vi "Fc_to_define_CSstatus.vi"(6 "Class TCP in":T1, 7 "CS enable":bool, 8 "error in (no error)":errorcluster, 10 "CS enable":refnum<vi>, 11 "# Control?":refnum<vi>) -> (0 "error out":errorcluster, 3 "Class TCP out":T1)   [LabVIEW 2021]
doc: "This function defines the current status of the control system."
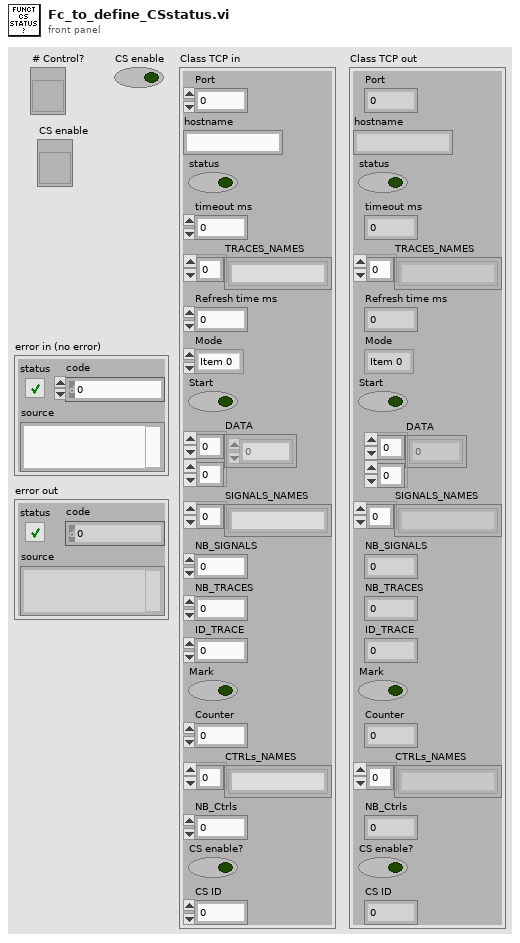
[diagram p1: front panel]
types:
  T1 = cluster{"Port":i32, "hostname":string, "status":bool, "timeout ms":i32, "TRACES_NAMES":string[], "Refresh time ms":i32, "Mode":enum32{"Item 0", "Item 1"}, "Start":bool, "DATA":sgl[][], "SIGNALS_NAMES":string[], "NB_SIGNALS":i32, "NB_TRACES":i32, "ID_TRACE":i32, "Mark":bool, "Counter":i32, "CTRLs_NAMES":string[], "NB_Ctrls":i32, "CS enable?":bool, "CS ID":i32}
  T2 = cluster{"TRACE_SIZE":i32, "CS_ID":i32, "TRACE ID":i32, "CMD":i32, "DATA(M)":i32}
  T3 = cluster{"timeout ms":i32, "remote port":u16, "Address":string}
  T4 = cluster{"SIZE":i32, " TRACE DATA":sgl[], "TRACE_SIZE":i32, "NB_TRACES":i32, "NB_TRACED_SIGNALS":i32, "NAMES TRACED SIGNALS":string[], "NAMES TRACES":string[], "CS STATUS":i32, "NB_CSs":i32, "NAMES CSs":string[], "DATA (M)":sgl[], "CMD":i32}
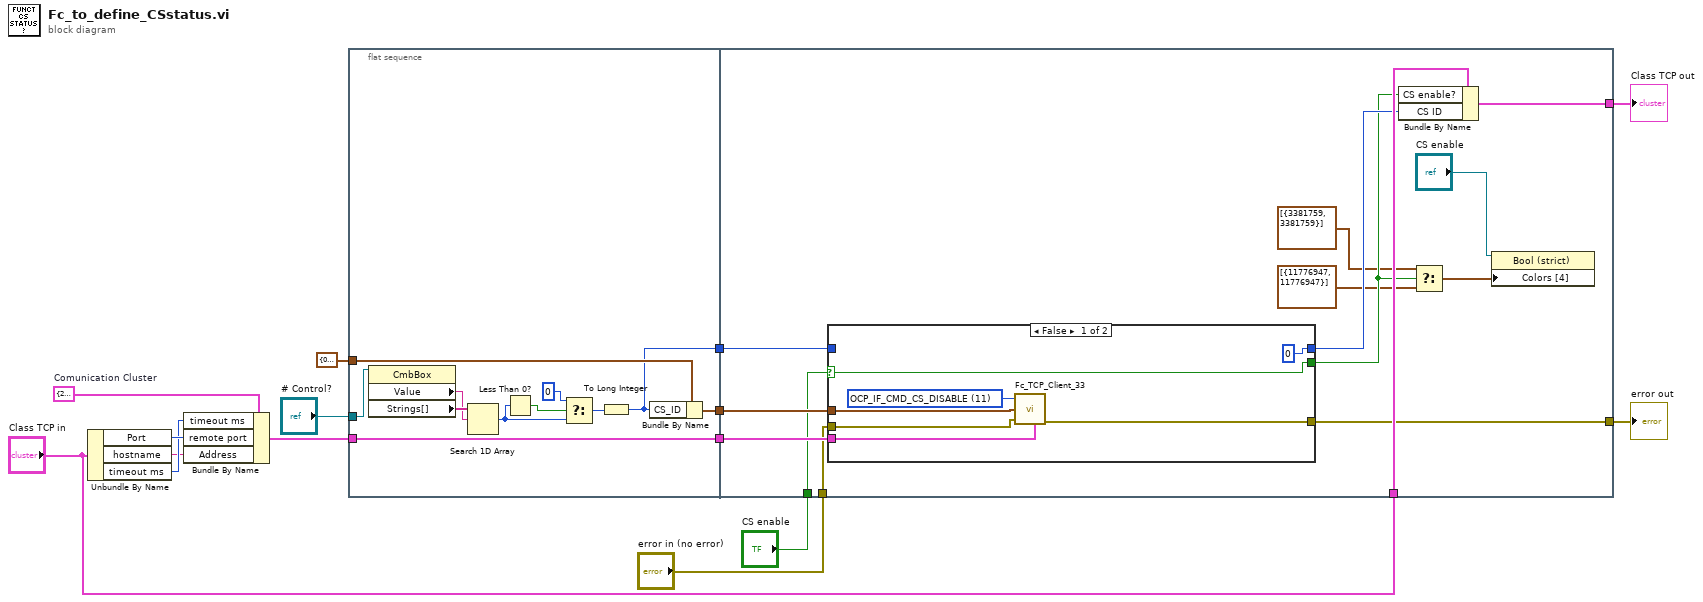
[diagram p0: block diagram]
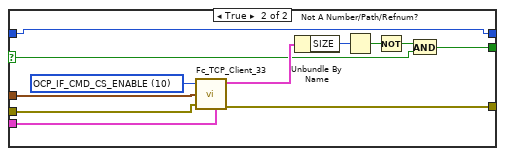
[diagram p2: hidden frame]
diagram:
  w12 = T3 {"timeout ms"=2000, "remote port"=8085, "Address"="127.0.0.1"}  # Comunication Cluster
  n1 = Unbundle By Name("Class TCP in") -> ("Port"=w6:i32, "hostname"=w4:string, "timeout ms"=w5:i32)
  n2 = Bundle By Name(cluster=w12, "timeout ms"=w5, "remote port"=w6, "Address"=w4) -> (w3:T3)
  n3 = flat-sequence {
    tunnel: T2 {"TRACE_SIZE"=0, "CS_ID"=0, "TRACE ID"=0, "CMD"=0, "DATA(M)"=0} ("Input Cluster") -> [w24]
    tunnel: w3 -> [w23]
    tunnel: [w23] -> w15
    tunnel: [w22] -> w14
    tunnel: [w17] -> w13
    tunnel: "# Control?" -> [w16]
    tunnel: w15 -> [w39]
    tunnel: w14 -> [w40]
    tunnel: "Class TCP in" -> [w38]
    tunnel: [w37] -> w7
    tunnel: w13 -> [w36]
    tunnel: "error in (no error)" -> [w30]
    tunnel: [w29] -> w10
    tunnel: "CS enable" -> [w28]
    frame #0 {
      n4 = property on="Property Node" class="CmbBox"(reference=w16) -> ("Value"=w25:string, "Strings[]"=w26:string[])  [unwired: 1 in, 2 out]
      n5 = Search 1D Array(1D array=w26, element=w25) -> (index of element=w20:i32)  [unwired: 1 in]
      n6 = Less Than 0?(x=w20) -> (x < 0?=w21:bool)
      n7 = Select(t=0, s=w21, f=w20) -> (s? t:f=w18:i32)
      n8 = To Long Integer(number=w18) -> (32bit integer=w17:i32)
      n9 = Bundle By Name(cluster=w24, "CS_ID"=w17) -> (w22:T2)
    }
    frame #1 {
      n10 = case shown="False" w28 {
        selector: w28 -> [w43 w54]
        tunnel: w39 -> [w47 w59]
        tunnel: w40 -> [w44 w56]
        tunnel: [w45 w57] -> w29
        tunnel: [w43 w53] -> w34
        tunnel: w36 -> [_ w52]
        tunnel: [0 w52] -> w35
        tunnel: w30 -> [w41 w48]
        frame False {
          w46 = 11 items=["OCP_IF_CMD_TRACE_READ", "OCP_IF_CMD_TRACE_RESET", "OCP_IF_CMD_TRACE_GET_SIZE", "OCP_IF_CMD_TRACE_SET_SIZE", "OCP_IF_CMD_TRACE_GET_NUMBER_SIGNALS", "OCP_IF_CMD_TRACE_GET_SIGNALS_NAMES", "OCP_IF_CMD_TRACE_GET_NUMBER_TRACES", "OCP_IF_CMD_TRACE_GET_TRACES_NAMES", "OCP_IF_CMD_TRACE_GET_ADDRESS", "OCP_IF_CMD_CS_STATUS", "OCP_IF_CMD_CS_ENABLE", "OCP_IF_CMD_CS_DISABLE", "OCP_IF_CMD_CS_CONTROLLER_IF", "OCP_IF_CMD_CS_HARDWARE_IF", "OCP_IF_CMD_CS_GET_NUMBER_CONTROLLERS", "OCP_IF_CMD_CS_GET_CONTROLLERS_NAMES", "OCP_IF_CMD_PLATFORM_ID", "OCP_IF_CMD_PLATFORM_IF", "OCP_IF_CMD_OPIL_UPDATE_MEASUREMENTS", "OCP_IF_CMD_OPIL_UPDATE_SIM_DATA", "OCP_IF_CMD_OPIL_RUN_CONTROL", "OCP_IF_CMD_OPIL_INITIALIZE_CONTROL", "OCP_IF_CMD_OPIL_GET_CONTROL", "OCP_IF_CMD_OPIL_GET_CONTROLLER_DATA", "OCP_IF_CMD_END"] ("CMD")
          n11 = call "Fc_TCP_Client_33.vi"("CMD"=w46, "Input Cluster"=w44, "error in (no error)"=w41, "Comunication Cluster"=w47) -> ("error out"=w45:errorcluster)  [unwired: 4 in, 2 out]
        }
        frame True {
          w58 = 10 items=["OCP_IF_CMD_TRACE_READ", "OCP_IF_CMD_TRACE_RESET", "OCP_IF_CMD_TRACE_GET_SIZE", "OCP_IF_CMD_TRACE_SET_SIZE", "OCP_IF_CMD_TRACE_GET_NUMBER_SIGNALS", "OCP_IF_CMD_TRACE_GET_SIGNALS_NAMES", "OCP_IF_CMD_TRACE_GET_NUMBER_TRACES", "OCP_IF_CMD_TRACE_GET_TRACES_NAMES", "OCP_IF_CMD_TRACE_GET_ADDRESS", "OCP_IF_CMD_CS_STATUS", "OCP_IF_CMD_CS_ENABLE", "OCP_IF_CMD_CS_DISABLE", "OCP_IF_CMD_CS_CONTROLLER_IF", "OCP_IF_CMD_CS_HARDWARE_IF", "OCP_IF_CMD_CS_GET_NUMBER_CONTROLLERS", "OCP_IF_CMD_CS_GET_CONTROLLERS_NAMES", "OCP_IF_CMD_PLATFORM_ID", "OCP_IF_CMD_PLATFORM_IF", "OCP_IF_CMD_OPIL_UPDATE_MEASUREMENTS", "OCP_IF_CMD_OPIL_UPDATE_SIM_DATA", "OCP_IF_CMD_OPIL_RUN_CONTROL", "OCP_IF_CMD_OPIL_INITIALIZE_CONTROL", "OCP_IF_CMD_OPIL_GET_CONTROL", "OCP_IF_CMD_OPIL_GET_CONTROLLER_DATA", "OCP_IF_CMD_END"] ("CMD")
          n12 = call "Fc_TCP_Client_33.vi"("CMD"=w58, "Input Cluster"=w56, "error in (no error)"=w48, "Comunication Cluster"=w59) -> ("Output cluster"=w55:T4, "error out"=w57:errorcluster)  [unwired: 4 in, 1 out]
          n13 = Unbundle By Name(w55) -> ("SIZE"=w51:i32)
          n14 = Not A Number/Path/Refnum?(number/path/refnum=w51) -> (NaN/Path/Refnum?=w50:bool)
          n15 = Not(x=w50) -> (.not. x?=w49:bool)
          n16 = And(x=w49, y=w54) -> (x .and. y?=w53:bool)
        }
      }
      n17 = Bundle By Name(cluster=w38, "CS enable?"=w34, "CS ID"=w35) -> (w37:T1)
      n18 = Select(t=cluster{u32, u32}[] [{3381759, 3381759}] ("Colors [4]"), s=w34, f=cluster{u32, u32}[] [{11776947, 11776947}] ("Colors [4]")) -> (s? t:f=w33:cluster{u32, u32}[])
      n19 = property on="Property Node" class="Bool (strict)"(reference="CS enable", "Colors [4]"=w33) -> ()  [unwired: 1 in, 2 out]
    }
  }
  "error out" <- w10
  "Class TCP out" <- w7
